vi "setFPGA.vi"(10 "FPGA":refnum<class "FPGA.lvclass">, 11 "ModbusRxDataFIFO in":refnum<class "ModbusRxDataFIFO.lvclass">) -> (3 "ModbusRxDataFIFO out":refnum<class "ModbusRxDataFIFO.lvclass">)   [LabVIEW 2016, in "ModbusRxDataFIFO.lvclass"]
uses:
  ModbusRxDataFIFO.lvclass
  FPGA/FPGA.lvclass
  ModbusRxDataFIFO.lvclass/ModbusRxDataFIFO.ctl
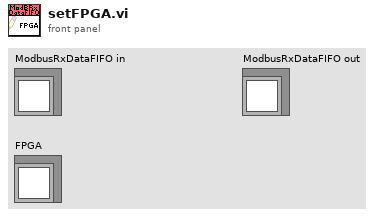
[diagram p1: front panel]
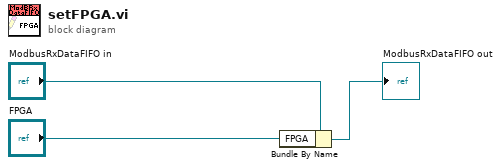
[diagram p0: block diagram]
diagram:
  n1 = Bundle By Name(cluster="ModbusRxDataFIFO in", "FPGA"="FPGA") -> (→"ModbusRxDataFIFO out":refnum<class "ModbusRxDataFIFO.lvclass">)
